vi "GOOP_ClassTool.vi"(0 "ClassRef":refnum<vi>, 5 "Error In":errorcluster) -> (19 "Error Out":errorcluster)   [LabVIEW 2014]
uses:
  <resource>/Framework/Providers/Open_GDS/ClassProviders/Common/ScriptingFunctions/Scripting_ConnectorPanePatternType.ctl
  <vilib>/regexp/Match Regular Expression.xnode
panel:
  out "ReasonWhyParentClassCan'tBeCreated 2":string
  in  "SelectAll":bool
  in  "ClassesCancel":bool
  in  "ClassesOK":bool
  in  "Classes":i32[](listbox)
  in  "MoreClasses":bool
  in  "Class(es)":u16(ring) items=["Oven", "-", "Equipment", "EquipmentVisitor", "GetCostVisitor", "Laser", "Oven", "PrintVisitor", "Rig"]
  in  "Tab":enum32{"CP", "ClassControlName", "Interface"}(tab)
  in  "ApplyCP":bool
  in  "CP2":u16(ring) caption="To" items=["4x4x4", "5x6x5", "6x8x6"]
  out "CP1":T1 caption="From" items=["4x4x4", "5x6x5", "6x8x6"]
  out "ClassNameOut":string
  out "ClassNameIn":string
  in  "ClassControlName":string(combo) caption="New names of class controls and indicators"
  in  "UpdateClassControlNames":bool
  in  "InterfaceToCreate":u16(ring) items=["Create a parent class based on some of my methods of my class: Oven", "Create an Interface(By VI Server) based on some of my methods of my class: Oven", "Create an Interface and Adaptor class based on some of my methods of my class: Oven"]
  out "InterfaceOptionTab":enum32{"Parent", "Adapter"}(tab)
  out "ReasonWhyParentClassCan'tBeCreated":string
  in  "CreateClassAndMethods":bool
  in  "ParentFolder":path
  in  "ParentClassName":string
  in  "ParentClass":u16(ring) items=["", "Equipment", "EquipmentVisitor", "GetCostVisitor", "Laser", "PrintVisitor", "Rig"]
  out "MyClassName(ParentClass)":string
  in  "MyClassMethods":i32[](listbox) caption="Class methods to add in the Interface class"
  out "Parent/InterafaceImage":u16(ring)
  out "MyClassName(InteraceClass)":string
  in  "InterfaceClassName 2":string
  in  "InterfaceFolder 2":path
  in  "Parent Methods":i32(listbox)
  in  "MyClassMethods(Interface)":i32[](listbox) caption="Class methods"
  in  "InterfaceClassName":string
  in  "InterfaceClass":u16(ring) items=["", "AbstractEdge", "Actor", "Last Ack", "Launch Nested Actor Msg", "Message", "Message Dequeuer", "Message Enqueuer", "Message Priority Queue", "Message Queue", "Stop Msg", "Actor1_BasicNoLib_G4_4.0.0", "Actor1_BasicNoLib_N_4.0.0", "Actor1_Basic_G4_4.0.0", "Actor1_Basic_N_4.0.0", "Actor1_GUI_G4_4.0.0", "StartMeasurement_Msg", "Actor1_GUI_N_4.0.0", "StartMeasurement_Msg", "AnotherClass", "ArrowHead", "Base", "BaseTemplate", "BaseTemplate_4x4x4", "BentStyle", "ByViServerInterfaceTemplate_4x4x4", "ByViServerInterfaceTemplate_6x8x6", "CallEdge", "ClassDiagramGraph", "ClassReader", "ClassReaderGOOP300", "ClassReaderGOOP400", "ClassReaderNative", "ClassRelationshipEdge", "ClassWriter", "ClassWriterGOOP300", "ClassWriterGOOP400", "ClassWriterNative", "DemoClass1", "DemoSubClass1", "DemoSubClass2", "DemoSubSubClass1", "Direction", "G4BaseTemplate_Simple_4x4x4", "G4BaseTemplate_Simple_6x8x6", "G4BaseTemplate_Singleton_4x4x4", "G4BaseTemplate_Singleton_6x8x6", "G4InterfaceTemplate_4x4x4", "G4InterfaceTemplate_6x8x6", "G4SubTemplate_Simple_4x4x4", "G4SubTemplate_Simple_6x8x6", "G4SubTemplate_Singleton_4x4x4", "G4SubTemplate_Singleton_6x8x6", "GOOP4_Base", "GOOP4_Sub", "GeneralPathEdge", "Graph", "Graphics", "Grid", "Interface1", "Leaf", "LineStyle", "Map", "Message_4.0.0", "MultiLineString", "NativeBaseTemplate", "NativeBaseTemplate_4x4x4", "NativeSubTemplate", "NativeSubTemplate_4x4x4", "NoteEdge", "Object", "Scripting", "SegmentedLineEdge", "SequenceDiagramGraph", "SingletonTemplate", "StateDiagramGraph", "StateReverse", "StateTransitionEdge", "Sub", "SubTemplate", "SubTemplate_4x4x4", "UmlEditor", "UseCaseDiagramGraph"]
  in  "InterfaceFolder":path
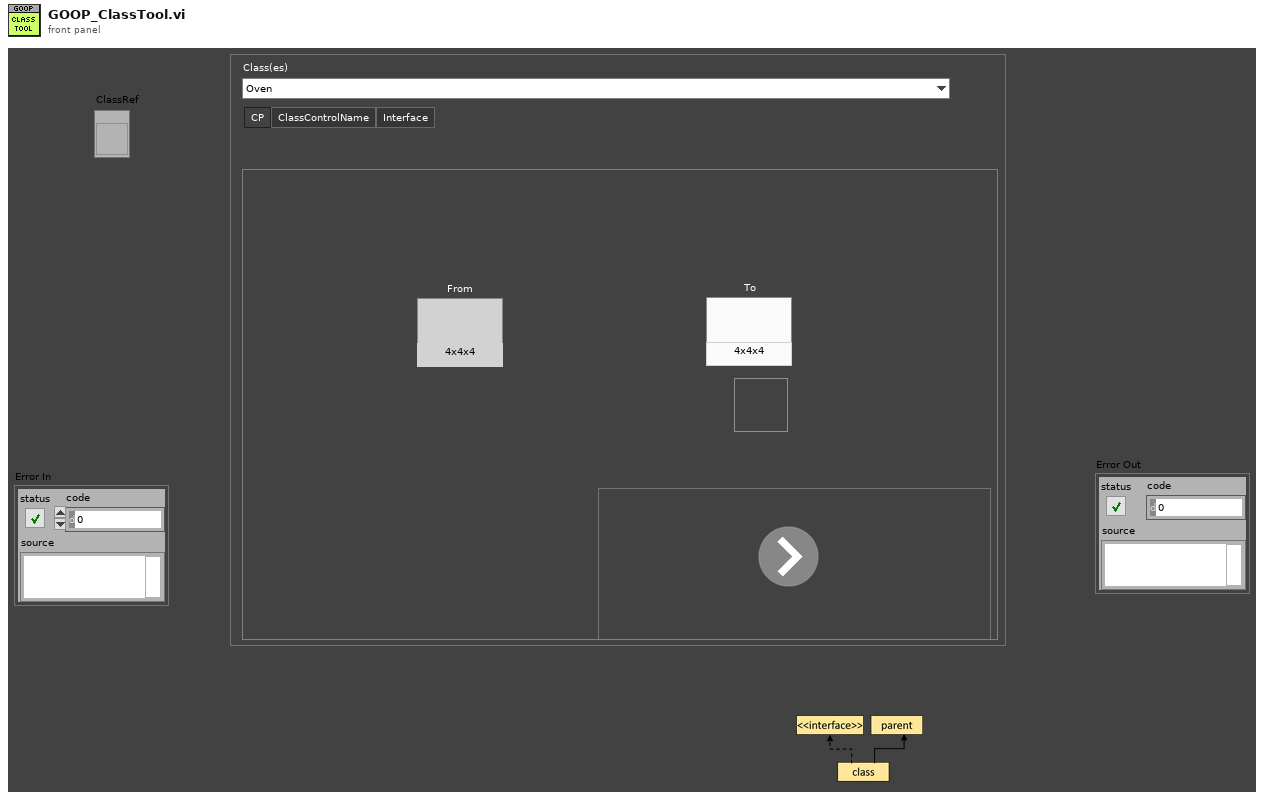
[diagram p1: front panel]
types:
  T1 = typedef "Scripting_ConnectorPanePatternType.ctl" = u16
  T2 = cluster{"Classes":refnum<vi>[], "Selected":i32[], "DropDownClasses":refnum<vi>[], "Interfaces":refnum<vi>[], "Methods":refnum<vi>[], "ParentClassIdx":i32}
  T3 = enum32{"Invalid", "Default", "Floating", "Floating/Auto-Hide", "Modal"}
  T4 = enum8{"Enabled", "Disabled", "Disabled and Grayed Out"}
  T5 = enum32{"invalid scope", "public", "private", "protected", "community"}
  T6 = typedef "GDSLvCLass_ClassSettingsType.ctl" = cluster{"ClassProviderName":string, "ClassTemplateUsed":string, "ClassTemplateVersion":string, "ClassDescription":string, "PlugIns":T7[], "ConnectorPanePattern":string}
  T7 = typedef "GDSLvClass_PlugIn.ctl" = cluster{"Type":T8, "ID":string, "Version":string, "Path":path, "Name":string, "Data":variant}
  T8 = typedef "GDSLvClass_PlugInTypes.ctl" = enum16{"DesignPattern", "MethodTypes"}
  T9 = cluster{"result string":string, "ClassRef":refnum<vi>}
  T10 = cluster{"result string":string, "ClassRef":refnum<vi>}[]
  T11 = typedef "lveventtype.ctl" = enum32{"Null", "Timeout", "Annotation Menu Selection", "Annotation Menu Selection?", "App Instance Close", "App Instance Close?", "Autoscale Range Change", "Bookmark Info Change", "Cell Edit", "Cell Edit?", "Cursor Grab", "Cursor Grab?", "Cursor Menu Selection", "Cursor Menu Selection?", "Cursor Move", "Cursor Release", "Data Change", "Direction Change", "Display State Change", "Drag Ended", "Drag Enter", "Drag Leave", "Drag Over", "Drag Source Update", "Drag Starting", "Drag Starting?", "Drop", "Exec State Change", "Key Down", "Key Down?", "Key Repeat", "Key Repeat?", "Key Up", "Listbox Double Click", "Menu Activation?", "Menu Selection (App)", "Menu Selection? (App)", "Menu Selection (User)", "Mouse Down", "Mouse Down?", "Mouse Enter", "Mouse Leave", "Mouse Move", "Mouse Up", "Mouse Wheel", "NI Security User Change (App)", "Pane Size", "Panel Close", "Panel Close?", "Panel Resize", "Plot Attribute Change", "Scale Range Change", "Shortcut Menu Activation?", "Shortcut Menu Selection (App)", "Shortcut Menu Selection? (App)", "Shortcut Menu Selection (User)", "Tree Double Click", "Tree Drag", "Tree Drag?", "Tree Drop", "Tree Drop?", "Tree Item Close", "Tree Item Close?", "Tree Item Open", "Tree Item Open?", "User Event", "Value Change"}
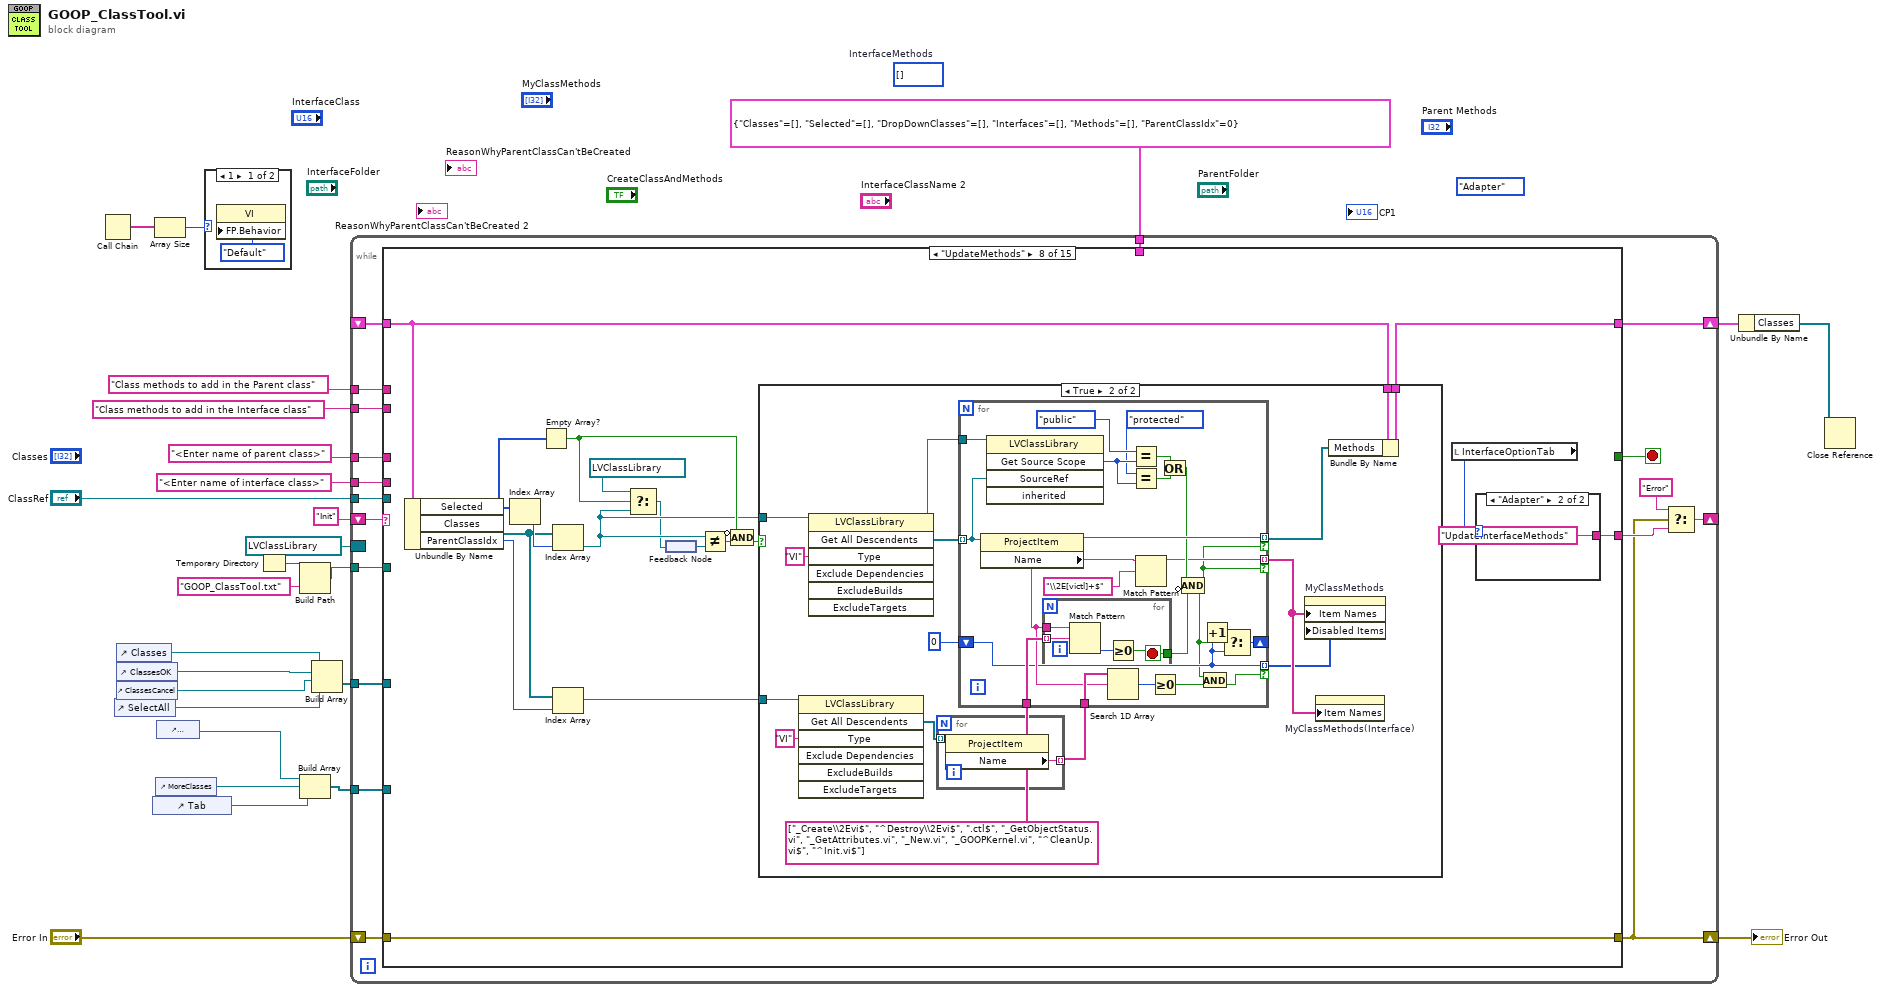
[diagram p0: block diagram]
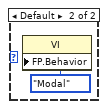
[diagram p2: hidden frame]
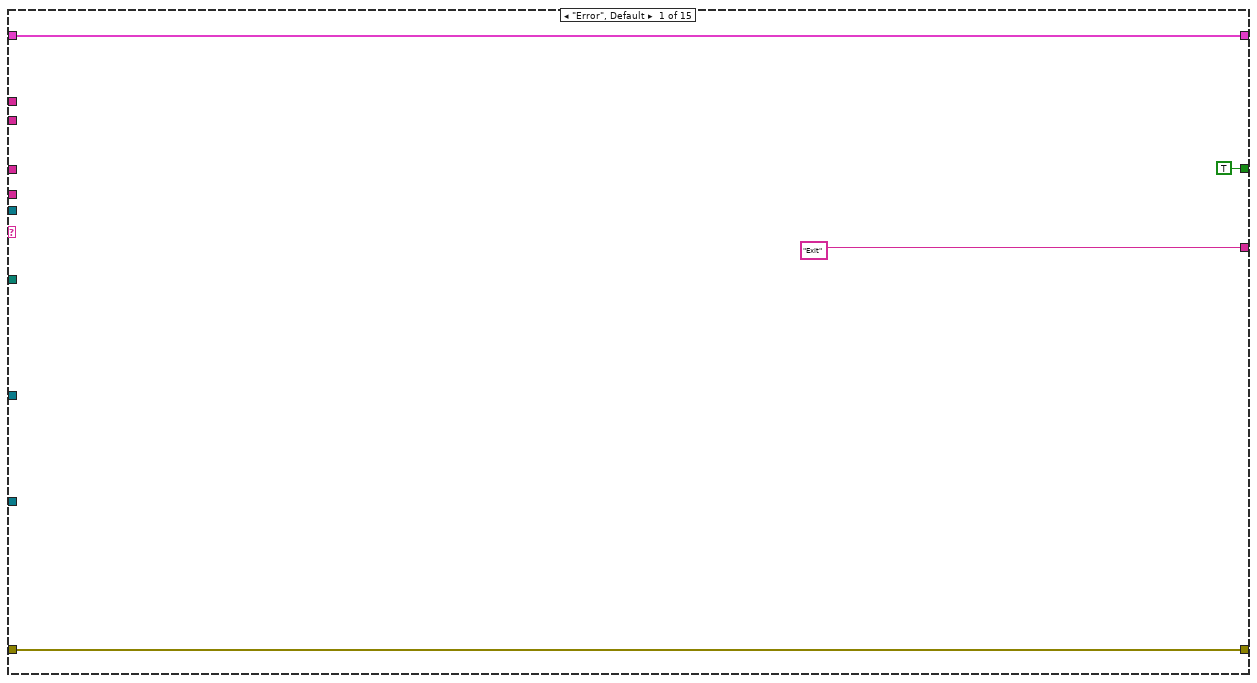
[diagram p3: hidden frame]
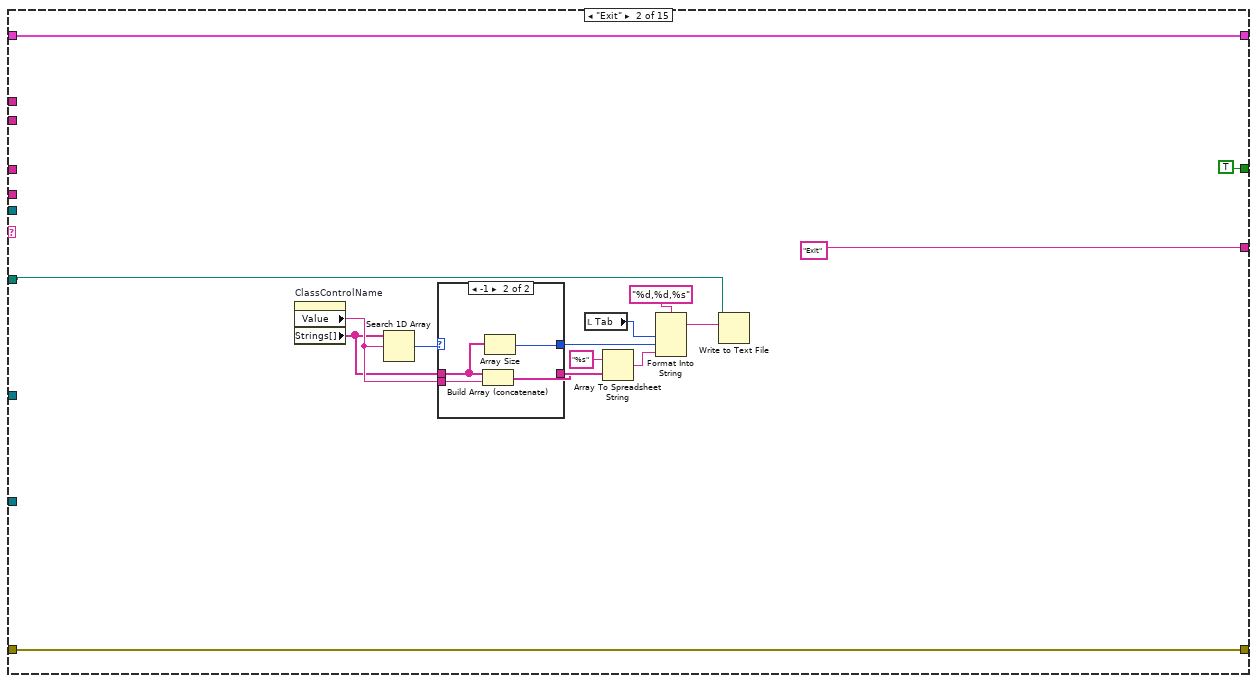
[diagram p4: hidden frame]
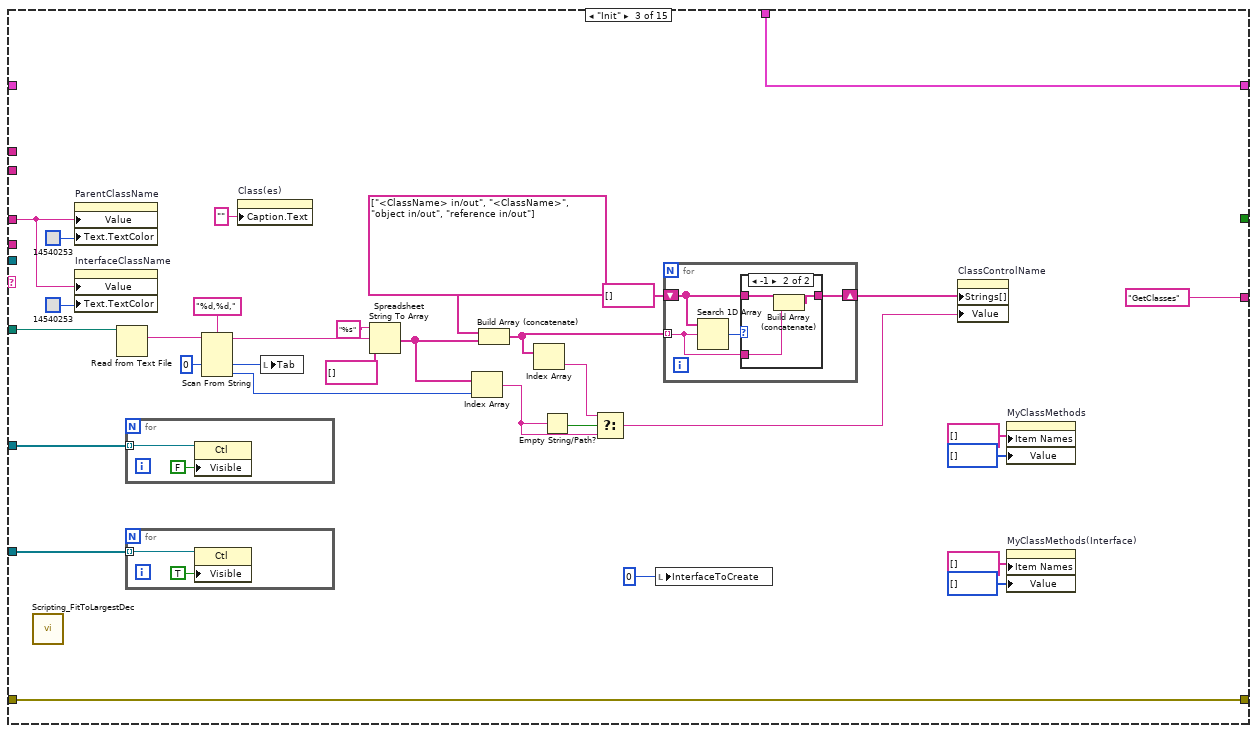
[diagram p6: hidden frame]
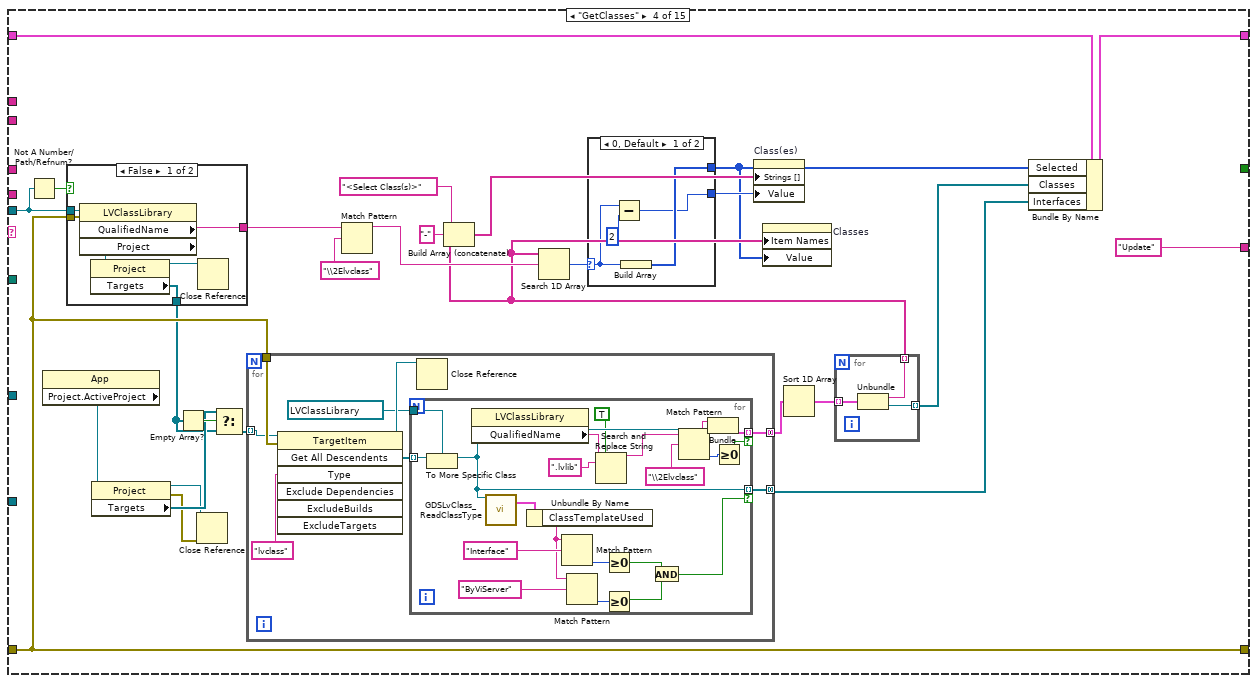
[diagram p8: hidden frame]
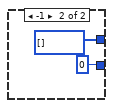
[diagram p9: hidden frame]
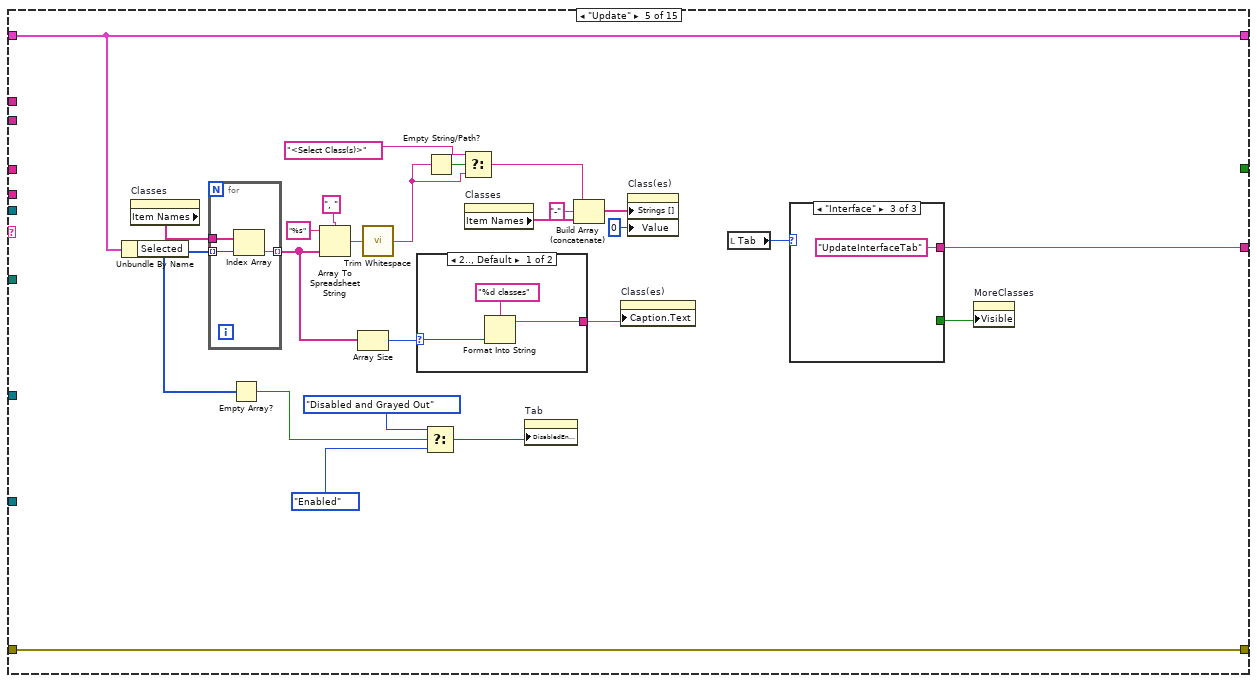
[diagram p11: hidden frame]
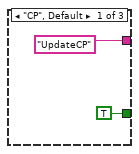
[diagram p12: hidden frame]
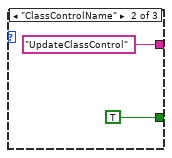
[diagram p13: hidden frame]
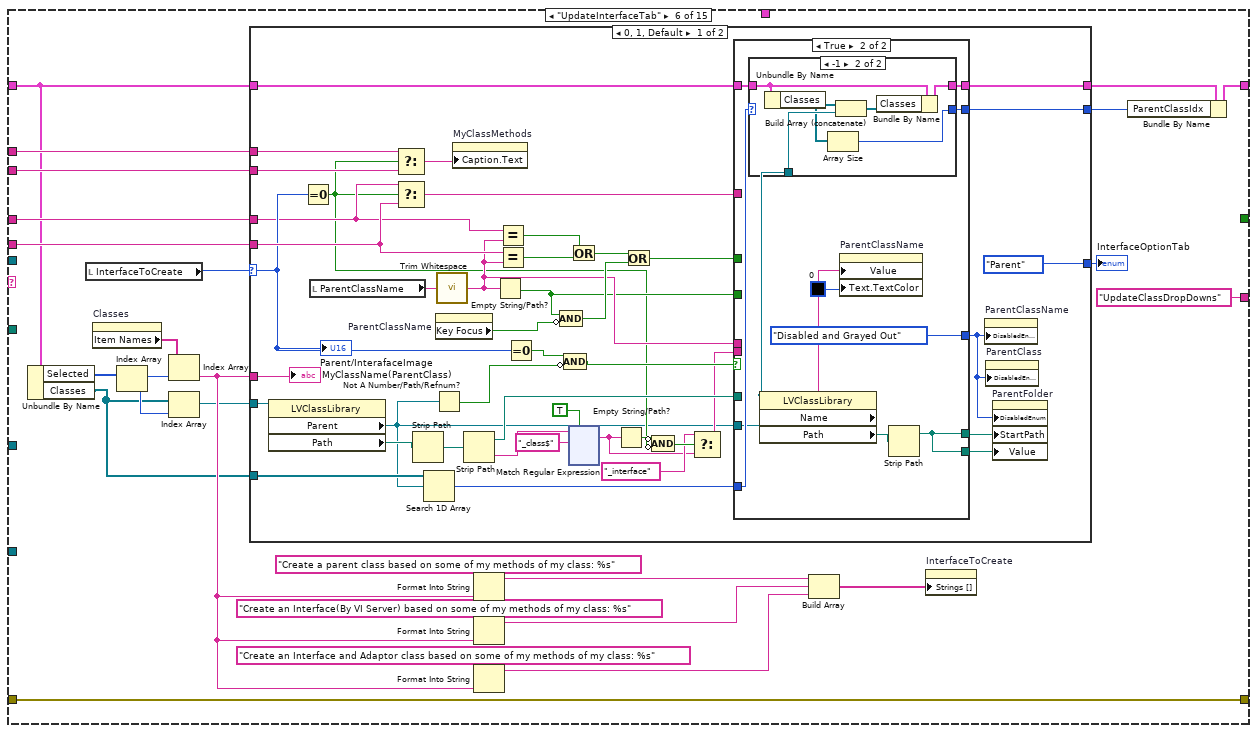
[diagram p15: hidden frame]
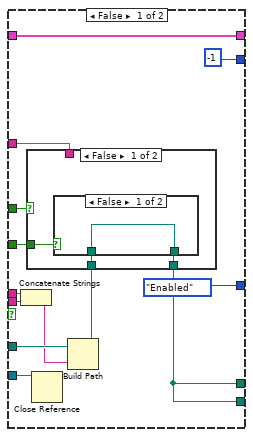
[diagram p16: hidden frame]
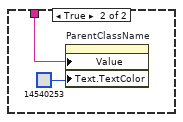
[diagram p18: hidden frame]
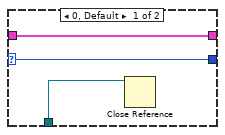
[diagram p19: hidden frame]
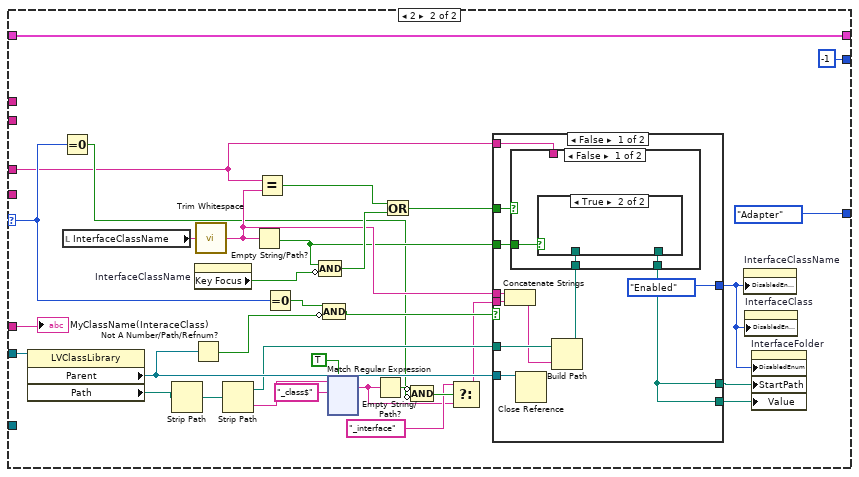
[diagram p20: hidden frame]
diagram:
  (unwired) enum32{"Parent", "Adapter"}."Adapter" ("InterfaceOptionTab")
  (unwired) i32[] []  # InterfaceMethods
  n1 = Call Chain() -> (call chain=w2:string[])
  n2 = control-ref of="SelectAll"() -> (w14:refnum<vi>)
  n3 = control-ref of="Classes"() -> (w23:refnum<vi>)
  n4 = control-ref of="ClassesOK"() -> (w22:refnum<vi>)
  n5 = control-ref of="ClassesCancel"() -> (w21:refnum<vi>)
  n6 = control-ref of="Tab"() -> (w18:refnum<vi>)
  n7 = Array Size(array=w2) -> (size(s)=w1:i32)
  n8 = control-ref of="MoreClasses"() -> (w19:refnum<vi>)
  n9 = control-ref of="Class(es)"() -> (w13:refnum<vi>)
  n10 = case shown="1" w1 {
    frame 1 {
      n11 = property class="VI"("FP.Behavior"=T3."Default" ("Front Panel Window:Behavior")) -> ()  [unwired: 2 in, 2 out]
    }
    frame Default {
      n12 = property class="VI"("FP.Behavior"=T3."Modal" ("Front Panel Window:Behavior")) -> ()  [unwired: 2 in, 2 out]
    }
  }
  n13 = Temporary Directory() -> (w9:path)
  n14 = Build Path(base path=w9, name or relative path="GOOP_ClassTool.txt") -> (appended path=w8:path)
  n15 = Build Array(w13, w19, w18) -> (w17:refnum<vi>[])
  n16 = Build Array(w23, w22, w21, w14) -> (w20:refnum<vi>[])
  n17 = while {
    shift-right: [w41] -> w24
    shift-left: "Error In" -> [w46]
    shift-right: [w44] -> _
    shift-left: "Init" -> [w45]
    shift-right: [w40] -> w12
    shift-left: _ -> [w39]
    tunnel: w20 -> [w38]
    tunnel: w17 -> [w37]
    tunnel: "ClassRef" -> [w36]
    tunnel: T2 {"Classes"=[], "Selected"=[], "DropDownClasses"=[], "Interfaces"=[], "Methods"=[], "ParentClassIdx"=0} -> [w35]
    tunnel: w8 -> [w34]
    tunnel: "<Enter name of parent class>" ("ParentClassName") -> [w32]
    tunnel: "<Enter name of interface class>" ("ParentClassName") -> [w31]
    tunnel: "Class methods to add in the Parent class" ("Caption.Text") -> [w30]
    tunnel: "Class methods to add in the Interface class" ("Caption.Text") -> [w29]
    border: refnum<vi> refnum ("ClassRef") -> [_]
    stop <- w33 stop-if-true
    n18 = case shown="\"UpdateMethods\"" w45 {
      tunnel: w46 -> [w50 w65 w102 w125 w212 w238 w619 w688 w736 w766 w814 w973 w982 w1000 w1042]
      tunnel: [w50 w65 w102 w125 w212 w238 w619 w688 w736 w766 w814 w973 w981 w997 w1042] -> w41
      tunnel: ["Exit" "Exit" "GetClasses" "Update" w200 "UpdateClassDropDowns" "UpdateMethods" w676 _ _ w815 "Update" "Exit" "Exit" _] -> w42
      tunnel: [w48 w63 w98 w128 w201 w227 w618 w684 w737 w765 w816 w974 w983 w1003 w1041] -> w40
      tunnel: w39 -> [w48 w63 _ w141 w201 w226 w616 w685 w737 w765 w811 w976 w983 w1003 w1041]
      tunnel: w38 -> [_ _ w101 _ _ _ _ _ _ _ w813 _ _ _ _]
      tunnel: w37 -> [_ _ w100 _ _ _ _ _ _ _ w812 _ _ _ _]
      tunnel: w36 -> [_ _ _ w124 _ _ _ _ _ _ _ _ _ _ _]
      tunnel: w35 -> [_ _ w98 _ _ _ _ _ _ _ _ _ _ _ _]
      tunnel: w34 -> [_ w52 w90 _ _ _ _ _ _ _ _ _ _ _ _]
      tunnel: [TRUE TRUE _ _ _ _ _ _ _ _ _ _ _ _ _] -> w33
      tunnel: w32 -> [_ _ w72 _ _ w237 _ _ _ _ w810 _ _ _ _]
      tunnel: w31 -> [_ _ _ _ _ w234 _ _ _ _ w808 _ _ _ _]
      tunnel: w30 -> [_ _ _ _ _ w230 _ _ _ _ _ _ _ _ _]
      tunnel: w29 -> [_ _ _ _ _ w229 _ _ _ _ _ _ _ _ _]
      frame "Error", Default {
      }
      frame "Exit" {
        n19 = property on="ClassControlName" class="CmbBox"() -> ("Value"=w57:string, "Strings[]"=w56:string[])  [unwired: 2 in, 2 out]
        n20 = Search 1D Array(1D array=w56, element=w57) -> (index of element=w53:i32)  [unwired: 1 in]
        n21 = case shown="-1" w53 {
          selector: w53 -> [w67 _]
          tunnel: [w67 w69] -> w54
          tunnel: w56 -> [w66 w70]
          tunnel: w57 -> [_ w71]
          tunnel: [w66 w68] -> w60
          frame 0, Default {
          }
          frame -1 {
            n22 = Build Array (concatenate)(w70, w71) -> (w68:string[])
            n23 = Array Size(array=w70) -> (size(s)=w69:i32)
          }
        }
        n24 = local read "Tab"() -> (w62:enum32{"CP", "ClassControlName", "Interface"})
        n25 = Array To Spreadsheet String(array=w60, 3:"%s" ("format string")) -> (spreadsheet string=w59:string)  [unwired: 1 in]
        n26 = Format Into String(format string="%d,%d,%s", w62, w54, w59) -> (resulting string=w61:string)  [unwired: 2 in, 1 out]
        n27 = Write to Text File(file (use dialog)=w52, text=w61) -> ()  [unwired: 2 in, 3 out]
      }
      frame "Init" {
        n28 = call <resource>:"Scripting_FitToLargestDec.vi"() -> ()  [unwired: 6 in, 2 out]
        n29 = property on="ParentClassName" class="Str"("Value"=w72, "Text.TextColor"=u32 14540253) -> ()  [unwired: 2 in, 2 out]
        n30 = property on="InterfaceClassName" class="Str"("Value"=w72, "Text.TextColor"=u32 14540253) -> ()  [unwired: 2 in, 2 out]
        n31 = Read from Text File(file (use dialog)=w90) -> (text=w97:string)  [unwired: 3 in, 3 out]
        n32 = for {
          tunnel: w101 -> [w115] mode=indexing
          n33 = property on="Property Node" class="Ctl"(reference=w115, "Visible"=FALSE) -> ()  [unwired: 1 in, 2 out]
        }
        n34 = for {
          tunnel: w100 -> [w113] mode=indexing
          n35 = property on="Property Node" class="Ctl"(reference=w113, "Visible"=TRUE) -> ()  [unwired: 1 in, 2 out]
        }
        n36 = Scan From String(format string="%d,%d,", input string=w97, default 1=0 ("default value 1")) -> (remaining string=w95:string, output 1=w88:i32, output 2=w86:i32)  [unwired: 3 in, 2 out]
        n37 = property on="Class(es)" class="Ring (strict)"("Caption.Text"="") -> ()  [unwired: 2 in, 2 out]
        n38 = local write "Tab"(w88) -> ()
        n39 = Spreadsheet String To Array(format string="%s", spreadsheet string=w95, array type (2D Dbl)=string[] []) -> (array=w87:string[])  [unwired: 1 in]
        n40 = Index Array(array=w87, index=w86) -> (element=w81:string)
        n41 = Build Array (concatenate)(string[] ["<ClassName> in/out", "<ClassName>", "object in/out", "reference in/out"] ("Strings []"), w87) -> (w84:string[])
        n42 = Index Array(array=w84) -> (element=w82:string)  [unwired: 1 in]
        n43 = Empty String/Path?(string/path=w81) -> (empty?=w83:bool)
        n44 = Select(t=w82, s=w83, f=w81) -> (s? t:f=w80:string)
        n45 = local write "InterfaceToCreate"(0) -> ()
        n46 = for {
          tunnel: w84 -> [w105] mode=indexing
          shift-right: [w104] -> w85
          shift-left: string[] [] -> [w106]
          n47 = Search 1D Array(1D array=w106, element=w105) -> (index of element=w107:i32)  [unwired: 1 in]
          n48 = case shown="-1" w107 {
            tunnel: w106 -> [w108 w111]
            tunnel: w105 -> [_ w110]
            tunnel: [w108 w109] -> w104
            frame 0, Default {
            }
            frame -1 {
              n49 = Build Array (concatenate)(w111, w110) -> (w109:string[])
            }
          }
        }
        n50 = property on="ClassControlName" class="CmbBox"("Strings[]"=w85, "Value"=w80) -> ()  [unwired: 2 in, 2 out]
        n51 = property on="MyClassMethods" class="LstBox (strict)"("Item Names"=string[] [], "Value"=i32[] [] ("MyClassMethods")) -> ()  [unwired: 2 in, 2 out]
        n52 = property on="MyClassMethods(Interface)" class="LstBox (strict)"("Item Names"=string[] [], "Value"=i32[] [] ("MyClassMethods")) -> ()  [unwired: 2 in, 2 out]
      }
      frame "GetClasses" {
        n53 = Not A Number/Path/Refnum?(number/path/refnum=w124) -> (NaN/Path/Refnum?=w123:bool)
        n54 = property class="App"() -> ("Project.ActiveProject"=w122:refnum<vi>)  [unwired: 2 in, 2 out]
        n55 = case shown="False" w123 {
          tunnel: [w154 _] -> w140
          tunnel: [w152 _] -> w121
          tunnel: w125 -> [w151 _]
          tunnel: w124 -> [w150 _]
          frame False {
            n56 = property class="LVClassLibrary"(reference=w150, error in=w151) -> ("QualifiedName"=w154:string, "Project"=w153:refnum<vi>)  [unwired: 2 out]
            n57 = property class="Project"(reference=w153) -> (reference out=w149:refnum<vi>, "Targets"=w152:refnum<vi>[])  [unwired: 1 in, 1 out]
            n58 = Close Reference(reference=w149) -> ()  [unwired: 1 in, 1 out]
          }
          frame True {
          }
        }
        n59 = property class="Project"(reference=w122) -> (reference out=w117:refnum<vi>, error out=w118:errorcluster, "Targets"=w133:refnum<vi>[])  [unwired: 1 in]
        n60 = Empty Array?(array=w121) -> (empty?=w134:bool)
        n61 = Close Reference(reference=w117, error in (no error)=w118) -> ()  [unwired: 1 out]
        n62 = Select(t=w133, s=w134, f=w121) -> (s? t:f=w132:refnum<vi>[])
        n63 = for {
          tunnel: [w163] -> w136 mode=concatenating
          tunnel: w125 -> [w162]
          tunnel: w132 -> [w161] mode=indexing
          tunnel: [w158] -> w116 mode=concatenating
          n64 = invoke class="TargetItem" method="Get All Descendents"(reference=w161, error in=w162, "Type"="lvclass") -> (reference out=w160:refnum<vi>, "All Descendents"=w164:refnum<vi>[])  [unwired: 4 in, 5 out]
          n65 = for {
            tunnel: w164 -> [w187] mode=indexing
            tunnel: [w181] -> w163 mode=indexing if=w184
            tunnel: refnum<vi> refnum ("ClassRef") -> [w176]
            tunnel: [w167] -> w158 mode=indexing if=w166
            n66 = To More Specific Class(target class=w176, reference=w187) -> (specific class reference=w167:refnum<vi>)  [unwired: 1 in, 1 out]
            n67 = property class="LVClassLibrary"(reference=w167) -> (reference out=w182:refnum<vi>, "QualifiedName"=w180:string)  [unwired: 1 in, 1 out]
            n68 = call <resource>:"GDSLvClass_ReadClassType.vi"("Class Refnum In"=w167) -> ("ClassSettings"=w173:T6)  [unwired: 16 in, 2 out]
            n69 = Unbundle By Name(w173) -> ("ClassTemplateUsed"=w170:string)
            n70 = Match Pattern(string=w170, regular expression="Interface") -> (offset past match=w171:i32)  [unwired: 1 in, 3 out]
            n71 = Match Pattern(string=w170, regular expression="ByViServer") -> (offset past match=w168:i32)  [unwired: 1 in, 3 out]
            n72 = Search and Replace String(replace all?=TRUE ("replace all? (F)"), input string=w180, search string=".lvlib" ("regular expression")) -> (result string=w179:string)  [unwired: 5 in, 3 out]
            n73 = Greater Or Equal To 0?(x=w171) -> (x >= 0?=w174:bool)
            n74 = Greater Or Equal To 0?(x=w168) -> (x >= 0?=w175:bool)
            n75 = And(x=w174, y=w175) -> (x .and. y?=w166:bool)
            n76 = Match Pattern(string=w179, regular expression="\\2Elvclass") -> (before substring=w183:string, offset past match=w185:i32)  [unwired: 1 in, 2 out]
            n77 = Bundle("result string"=w183, "ClassRef"=w182) -> (w181:T9)  [unwired: 1 in]
            n78 = Greater Or Equal To 0?(x=w185) -> (x >= 0?=w184:bool)
          }
          n79 = Close Reference(reference=w160) -> ()  [unwired: 1 in, 1 out]
        }
        n80 = Match Pattern(string=w140, regular expression="\\2Elvclass") -> (before substring=w131:string)  [unwired: 1 in, 3 out]
        n81 = Sort 1D Array(array=w136) -> (sorted array=w130:T10)
        n82 = for {
          tunnel: w130 -> [w157] mode=indexing
          tunnel: [w156] -> w127 mode=indexing
          tunnel: [w155] -> w129 mode=indexing
          n83 = Unbundle(w157) -> ("result string"=w155:string, "ClassRef"=w156:refnum<vi>)
        }
        n84 = Build Array (concatenate)("<Select Class(s)>" ("element"), "-" ("element"), w129) -> (w137:string[])
        n85 = Search 1D Array(1D array=w129, element=w131) -> (index of element=w120:i32)  [unwired: 1 in]
        n86 = case shown="0, Default" w120 {
          selector: w120 -> [w146 _]
          tunnel: [w143 0 ("Classes")] -> w135
          tunnel: [w145 i32[] [] ("Classes")] -> w119
          frame 0, Default {
            n87 = Subtract(x=w146, y=2) -> (x-y=w143:i32)
            n88 = Build Array(w146) -> (w145:i32[])
          }
          frame -1 {
          }
        }
        n89 = property on="Class(es)" class="Ring (strict)"("Strings []"=w137, "Value"=w135) -> ()  [unwired: 2 in, 2 out]
        n90 = property on="Classes" class="LstBox (strict)"("Item Names"=w129, "Value"=w119) -> ()  [unwired: 2 in, 2 out]
        n91 = Bundle By Name(cluster=w141, "Selected"=w119, "Classes"=w127, "Interfaces"=w116) -> (w128:T2)
      }
      frame "Update" {
        n92 = Unbundle By Name(w201) -> ("Selected"=w199:i32[])
        n93 = property on="Classes" class="LstBox (strict)"() -> ("Item Names"=w211:string[])  [unwired: 2 in, 2 out]
        n94 = for {
          tunnel: w199 -> [w223] mode=indexing
          tunnel: w211 -> [w222]
          tunnel: [w221] -> w188 mode=indexing
          n95 = Index Array(array=w222, index=w223) -> (element=w221:string)
        }
        n96 = Empty Array?(array=w199) -> (empty?=w198:bool)
        n97 = Array To Spreadsheet String(delimiter (Tab)=", ", array=w188, 3:"%s" ("format string")) -> (spreadsheet string=w208:string)
        n98 = Array Size(array=w188) -> (size(s)=w207:i32)
        n99 = call <vilib>:"Trim Whitespace.vi"("string"=w208) -> ("trimmed string"=w192:string)  [unwired: 1 in]
        n100 = case shown="2.., Default" w207 {
          selector: w207 -> [w220 _]
          tunnel: [w218 _] -> w206
          frame 2.., Default {
            n101 = Format Into String(format string="%d classes", w220) -> (resulting string=w218:string)  [unwired: 2 in, 1 out]
          }
          frame ..1 {
          }
        }
        n102 = Select(t=T4."Disabled and Grayed Out", s=w198, f=T4."Enabled" ("Disabled")) -> (s? t:f=w195:T4)
        n103 = Empty String/Path?(string/path=w192) -> (empty?=w194:bool)
        n104 = Select(t="<Select Class(s)>" ("element"), s=w194, f=w192) -> (s? t:f=w191:string)
        n105 = property on="Classes" class="LstBox (strict)"() -> ("Item Names"=w205:string[])  [unwired: 2 in, 2 out]
        n106 = property on="Tab" class="TabCtl (strict)"("DisabledEnum"=w195) -> ()  [unwired: 2 in, 2 out]
        n107 = Build Array (concatenate)(w191, "-" ("element"), w205) -> (w204:string[])
        n108 = property on="Class(es)" class="Ring (strict)"("Caption.Text"=w206) -> ()  [unwired: 2 in, 2 out]
        n109 = property on="Class(es)" class="Ring (strict)"("Strings []"=w204, "Value"=0 ("Classes")) -> ()  [unwired: 2 in, 2 out]
        n110 = local read "Tab"() -> (w190:enum32{"CP", "ClassControlName", "Interface"})
        n111 = case shown="\"Interface\"" w190 {
          tunnel: ["UpdateCP" "UpdateClassControl" "UpdateInterfaceTab"] -> w200
          tunnel: [TRUE TRUE _] -> w189
          frame "CP", Default {
          }
          frame "ClassControlName" {
          }
          frame "Interface" {
          }
        }
        n112 = property on="MoreClasses" class="Bool"("Visible"=w189) -> ()  [unwired: 2 in, 2 out]
      }
      frame "UpdateInterfaceTab" {
        n113 = Unbundle By Name(w226) -> ("Selected"=w248:i32[], "Classes"=w228:refnum<vi>[])
        n114 = local read "InterfaceToCreate"() -> (w235:u16)
        n115 = property on="Classes" class="LstBox (strict)"() -> ("Item Names"=w247:string[])  [unwired: 2 in, 2 out]
        n116 = Index Array(array=w248) -> (element=w232:i32)  [unwired: 1 in]
        n117 = Index Array(array=w247, index=w232) -> (element=w239:string)
        n118 = Index Array(array=w228, index=w232) -> (element=w231:refnum<vi>)
        n119 = case shown="0, 1, Default" w235 {
          selector: w235 -> [w278 w468]
          tunnel: w239 -> [w291 w448]
          tunnel: w237 -> [w266 w447]
          tunnel: [enum32{"Parent", "Adapter"}."Parent" ("InterfaceOptionTab") enum32{"Parent", "Adapter"}."Adapter" ("InterfaceOptionTab")] -> w236
          tunnel: w234 -> [w283 _]
          tunnel: w231 -> [w281 w472]
          tunnel: w230 -> [w265 _]
          tunnel: w229 -> [w264 _]
          tunnel: w228 -> [w254 _]
          tunnel: w226 -> [w251 w445]
          tunnel: [w250 w445] -> w225
          tunnel: [w249 -1 ("index of element")] -> w224
          frame 0, 1, Default {
            n120 = property class="LVClassLibrary"(reference=w281) -> ("Parent"=w253:refnum<vi>, "Path"=w275:path)  [unwired: 1 in, 2 out]
            n121 = Equal To 0?(x=w278) -> (x = 0?=w260:bool)
            n122 = local read "ParentClassName"() -> (w290:string)
            n123 = Select(t=w265, s=w260, f=w264) -> (s? t:f=w263:string)
            n124 = Select(t=w266, s=w260, f=w283) -> (s? t:f=w282:string)
            n125 = Strip Path(path=w275) -> (stripped path=w274:path)  [unwired: 1 out]
            n126 = Search 1D Array(1D array=w254, element=w253) -> (index of element=w252:i32)  [unwired: 1 in]
            n127 = Not A Number/Path/Refnum?(number/path/refnum=w253) -> (NaN/Path/Refnum?=w279:bool)
            n128 = property on="ParentClassName" class="Str"() -> ("Key Focus"=w289:bool)  [unwired: 2 in, 2 out]
            n129 = call <vilib>:"Trim Whitespace.vi"("string"=w290) -> ("trimmed string"=w268:string)  [unwired: 1 in]
            n130 = property on="MyClassMethods" class="LstBox (strict)"("Caption.Text"=w263) -> ()  [unwired: 2 in, 2 out]
            n131 = Strip Path(path=w274) -> (stripped path=w267:path, name=w271:string)
            n132 = Empty String/Path?(string/path=w268) -> (empty?=w262:bool)
            n133 = Equal?(x=w266, y=w268) -> (x = y?=w285:bool)
            n134 = Equal?(x=w283, y=w268) -> (x = y?=w286:bool)
            n135 = Equal To 0?(x=w278) -> (x = 0?=w277:bool)
            n136 = Compound Arithmetic op=AND(w262, invert w289) -> (w288:bool)
            n137 = Compound Arithmetic op=AND(w277, invert w279) -> (w276:bool)
            n138 = Or(x=w285, y=w286) -> (x .or. y?=w284:bool)
            n139 = xnode "Match Regular Expression"("input string"=w271, "regular expression"="_class$", "ignore case? (F)"=TRUE) -> ("whole match"=w257:string)  [unwired: 3 in, 4 out]
            n140 = Empty String/Path?(string/path=w257) -> (empty?=w261:bool)
            n141 = Or(x=w284, y=w288) -> (x .or. y?=w280:bool)
            n142 = Compound Arithmetic op=AND(invert w261, invert w260) -> (w259:bool)
            n143 = Select(t="_interface" ("regular expression"), s=w259, f=w257) -> (s? t:f=w256:string)
            n144 = case shown="True" w276 {
              tunnel: w282 -> [w418 _]
              tunnel: w253 -> [w416 w426]
              tunnel: w280 -> [w417 _]
              tunnel: [T4."Enabled" ("Disabled") T4."Disabled and Grayed Out" ("Disabled")] -> w255
              tunnel: [w410 w430] -> w273
              tunnel: [w410 w430] -> w272
              tunnel: w268 -> [w415 _]
              tunnel: w256 -> [w414 _]
              tunnel: w267 -> [w413 _]
              tunnel: w262 -> [w408 _]
              tunnel: w252 -> [_ w429]
              tunnel: w251 -> [w407 w428]
              tunnel: [w407 w427] -> w250
              tunnel: [-1 ("index of element") w425] -> w249
              frame False {
                n145 = Concatenate Strings(w415, w414) -> (w412:string)
                n146 = Close Reference(reference=w416) -> ()  [unwired: 1 in, 1 out]
                n147 = Build Path(base path=w413, name or relative path=w412) -> (appended path=w411:path)
                n148 = case shown="False" w417 {
                  tunnel: w418 -> [_ w423]
                  tunnel: w411 -> [w420 _]
                  tunnel: [w419 _] -> w410
                  tunnel: w408 -> [w421 _]
                  frame False {
                    n149 = case shown="False" w421 {
                      tunnel: w420 -> [w422 _]
                      tunnel: [w422 _] -> w419
                      frame False {
                      }
                      frame True {
                      }
                    }
                  }
                  frame True {
                    n150 = property on="ParentClassName" class="Str"("Value"=w423, "Text.TextColor"=u32 14540253) -> ()  [unwired: 2 in, 2 out]
                  }
                }
              }
              frame True {
                n151 = case shown="-1" w429 {
                  selector: w429 -> [w435 _]
                  tunnel: w428 -> [w437 w442]
                  tunnel: [w437 w443] -> w427
                  tunnel: w426 -> [w436 w440]
                  tunnel: [w435 w438] -> w425
                  frame 0, Default {
                    n152 = Close Reference(reference=w436) -> ()  [unwired: 1 in, 1 out]
                  }
                  frame -1 {
                    n153 = Unbundle By Name(w442) -> ("Classes"=w439:refnum<vi>[])
                    n154 = Array Size(array=w439) -> (size(s)=w438:i32)
                    n155 = Build Array (concatenate)(w439, w440) -> (w441:refnum<vi>[])
                    n156 = Bundle By Name(cluster=w442, "Classes"=w441) -> (w443:T2)
                  }
                }
                n157 = property class="LVClassLibrary"(reference=w426) -> ("Name"=w432:string, "Path"=w431:path)  [unwired: 1 in, 2 out]
                n158 = property on="ParentClassName" class="Str"("Value"=w432, "Text.TextColor"=u32 0) -> ()  [unwired: 2 in, 2 out]
                n159 = Strip Path(path=w431) -> (stripped path=w430:path)  [unwired: 1 out]
              }
            }
            n160 = property on="ParentClassName" class="Str"("DisabledEnum"=w255) -> ()  [unwired: 2 in, 2 out]
            n161 = property on="ParentClass" class="Ring (strict)"("DisabledEnum"=w255) -> ()  [unwired: 2 in, 2 out]
            n162 = property on="ParentFolder" class="Path"("DisabledEnum"=w255, "StartPath"=w273, "Value"=w272) -> ()  [unwired: 2 in, 2 out]
            "MyClassName(ParentClass)" <- w291
            "Parent/InterafaceImage" <- w278
          }
          frame 2 {
            n163 = property class="LVClassLibrary"(reference=w472) -> ("Parent"=w471:refnum<vi>, "Path"=w465:path)  [unwired: 1 in, 2 out]
            n164 = Equal To 0?(x=w468) -> (x = 0?=w454:bool)
            n165 = local read "InterfaceClassName"() -> (w476:string)
            n166 = Strip Path(path=w465) -> (stripped path=w464:path)  [unwired: 1 out]
            n167 = Not A Number/Path/Refnum?(number/path/refnum=w471) -> (NaN/Path/Refnum?=w469:bool)
            n168 = property on="InterfaceClassName" class="Str"() -> ("Key Focus"=w475:bool)  [unwired: 2 in, 2 out]
            n169 = call <vilib>:"Trim Whitespace.vi"("string"=w476) -> ("trimmed string"=w458:string)  [unwired: 1 in]
            n170 = Strip Path(path=w464) -> (stripped path=w457:path, name=w461:string)
            n171 = Empty String/Path?(string/path=w458) -> (empty?=w456:bool)
            n172 = Equal?(x=w447, y=w458) -> (x = y?=w446:bool)
            n173 = Equal To 0?(x=w468) -> (x = 0?=w467:bool)
            n174 = Compound Arithmetic op=AND(w456, invert w475) -> (w474:bool)
            n175 = Compound Arithmetic op=AND(w467, invert w469) -> (w466:bool)
            n176 = xnode "Match Regular Expression"("input string"=w461, "regular expression"="_class$", "ignore case? (F)"=TRUE) -> ("whole match"=w451:string)  [unwired: 3 in, 4 out]
            n177 = Empty String/Path?(string/path=w451) -> (empty?=w455:bool)
            n178 = Or(x=w446, y=w474) -> (x .or. y?=w470:bool)
            n179 = Compound Arithmetic op=AND(invert w455, invert w454) -> (w453:bool)
            n180 = Select(t="_interface" ("regular expression"), s=w453, f=w451) -> (s? t:f=w450:string)
            n181 = case shown="False" w466 {
              tunnel: w447 -> [w601 _]
              tunnel: w471 -> [w599 w613]
              tunnel: w470 -> [w600 _]
              tunnel: [T4."Enabled" ("Disabled") T4."Disabled and Grayed Out" ("Disabled")] -> w449
              tunnel: [w593 w608] -> w463
              tunnel: [w593 w608] -> w462
              tunnel: w458 -> [w598 _]
              tunnel: w450 -> [w597 _]
              tunnel: w457 -> [w596 _]
              tunnel: w456 -> [w591 _]
              frame False {
                n182 = Concatenate Strings(w598, w597) -> (w595:string)
                n183 = Close Reference(reference=w599) -> ()  [unwired: 1 in, 1 out]
                n184 = Build Path(base path=w596, name or relative path=w595) -> (appended path=w594:path)
                n185 = case shown="False" w600 {
                  tunnel: w601 -> [_ w606]
                  tunnel: w594 -> [w603 _]
                  tunnel: [w602 _] -> w593
                  tunnel: w591 -> [w604 _]
                  frame False {
                    n186 = case shown="True" w604 {
                      tunnel: w603 -> [w605 _]
                      tunnel: [w605 _] -> w602
                      frame False {
                      }
                      frame True {
                      }
                    }
                  }
                  frame True {
                    n187 = property on="InterfaceClassName" class="Str"("Value"=w606, "Text.TextColor"=u32 14540253) -> ()  [unwired: 2 in, 2 out]
                  }
                }
              }
              frame True {
                n188 = property class="LVClassLibrary"(reference=w613) -> (reference out=w614:refnum<vi>, "Name"=w610:string, "Path"=w609:path)  [unwired: 1 in, 1 out]
                n189 = property on="InterfaceClassName" class="Str"("Value"=w610, "Text.TextColor"=u32 0) -> ()  [unwired: 2 in, 2 out]
                n190 = Strip Path(path=w609) -> (stripped path=w608:path)  [unwired: 1 out]
                n191 = Close Reference(reference=w614) -> ()  [unwired: 1 in, 1 out]
              }
            }
            n192 = property on="InterfaceClassName" class="Str"("DisabledEnum"=w449) -> ()  [unwired: 2 in, 2 out]
            n193 = property on="InterfaceClass" class="Ring (strict)"("DisabledEnum"=w449) -> ()  [unwired: 2 in, 2 out]
            n194 = property on="InterfaceFolder" class="Path"("DisabledEnum"=w449, "StartPath"=w463, "Value"=w462) -> ()  [unwired: 2 in, 2 out]
            "MyClassName(InteraceClass)" <- w448
          }
        }
        "InterfaceOptionTab" <- w236
        n195 = Format Into String(format string="Create a parent class based on some of my methods of my class: %s", w239) -> (resulting string=w245:string)  [unwired: 2 in, 1 out]
        n196 = Format Into String(format string="Create an Interface(By VI Server) based on some of my methods of my class: %s", w239) -> (resulting string=w242:string)  [unwired: 2 in, 1 out]
        n197 = Format Into String(format string="Create an Interface and Adaptor class based on some of my methods of my class: %s", w239) -> (resulting string=w240:string)  [unwired: 2 in, 1 out]
        n198 = Build Array(w245, w242, w240) -> (w244:string[])
        n199 = property on="InterfaceToCreate" class="Ring (strict)"("Strings []"=w244) -> ()  [unwired: 2 in, 2 out]
        n200 = Bundle By Name(cluster=w225, "ParentClassIdx"=w224) -> (w227:T2)
      }
      frame "UpdateClassDropDowns" {
        n201 = local read "InterfaceToCreate"() -> (w620:u16)
        n202 = case shown="0, Default" w620 {
          tunnel: [w627 w664] -> w617
          tunnel: w616 -> [w623 w665]
          frame 0, Default {
            n203 = Unbundle By Name(w623) -> ("Classes"=w622:refnum<vi>[], "Selected"=w621:i32[])
            n204 = Index Array(array=w621) -> (element=w624:i32)  [unwired: 1 in]
            n205 = Index Array(array=w622, index=w624) -> (element=w629:refnum<vi>)
            n206 = property class="LVClassLibrary"(reference=w629) -> ("Name"=w631:string)  [unwired: 1 in, 2 out]
            n207 = for {
              tunnel: w622 -> [w645] mode=indexing
              tunnel: w631 -> [w640]
              shift-right: [w636] -> w627
              shift-left: refnum<vi>[] [] -> [w638]
              n208 = property class="LVClassLibrary"(reference=w645) -> (reference out=w637:refnum<vi>, "Name"=w643:string)  [unwired: 1 in, 1 out]
              n209 = Build Array(w643) -> (w642:string[])
              n210 = while {
                shift-right: [w652] -> w644
                shift-left: w637 -> [w658]
                shift-right: [w653] -> w641
                shift-left: w642 -> [w655]
                i -> [w650]
                stop <- w656 stop-if-true
                n211 = property class="LVClassLibrary"(reference=w658) -> (reference out=w651:refnum<vi>, error out=w657:errorcluster, "Parent"=w652:refnum<vi>)  [unwired: 1 in]
                n212 = case shown="1.." w650 {
                  tunnel: w651 -> [_ w659]
                  frame Default {
                  }
                  frame 1.. {
                    n213 = Close Reference(reference=w659) -> ()  [unwired: 1 in, 1 out]
                  }
                }
                n214 = property class="LVClassLibrary"(reference=w652, error in=w657) -> (error out=w656:errorcluster, "Name"=w654:string)  [unwired: 1 out]
                n215 = case shown="No Error" w656 {
                  tunnel: w655 -> [w662 w663]
                  tunnel: w654 -> [w661 _]
                  tunnel: [w660 w663] -> w653
                  frame No Error {
                    n216 = Build Array (concatenate)(w662, w661) -> (w660:string[])
                  }
                  frame Error {
                  }
                }
              }
              n217 = Close Reference(reference=w644) -> ()  [unwired: 1 in, 1 out]
              n218 = Search 1D Array(1D array=w641, element=w640) -> (index of element=w639:i32)  [unwired: 1 in]
              n219 = case shown="0, Default" w639 {
                tunnel: w638 -> [w646 w649]
                tunnel: w637 -> [_ w648]
                tunnel: [w646 w647] -> w636
                frame 0, Default {
                }
                frame -1 {
                  n220 = Build Array (concatenate)(w649, w648) -> (w647:refnum<vi>[])
                }
              }
            }
            n221 = for {
              tunnel: w627 -> [w635] mode=indexing
              tunnel: [w632] -> w628 mode=indexing
              n222 = property class="LVClassLibrary"(reference=w635) -> ("Name"=w633:string)  [unwired: 1 in, 2 out]
              n223 = Match Pattern(string=w633, regular expression="\\2Elvclass") -> (before substring=w632:string)  [unwired: 1 in, 3 out]
            }
            n224 = Build Array (concatenate)("" ("regular expression"), w628) -> (w626:string[])
            n225 = property on="ParentClass" class="Ring (strict)"("Strings []"=w626) -> ()  [unwired: 2 in, 2 out]
          }
          frame 1 {
            n226 = Unbundle By Name(w665) -> ("Interfaces"=w664:refnum<vi>[])
            n227 = for {
              tunnel: w664 -> [w672] mode=indexing
              tunnel: [w669] -> w668 mode=indexing
              n228 = property class="LVClassLibrary"(reference=w672) -> ("Name"=w670:string)  [unwired: 1 in, 2 out]
              n229 = Match Pattern(string=w670, regular expression="\\2Elvclass") -> (before substring=w669:string)  [unwired: 1 in, 3 out]
            }
            n230 = Build Array (concatenate)("" ("regular expression"), w668) -> (w667:string[])
            n231 = property on="ParentClass" class="Ring (strict)"("Strings []"=w667) -> ()  [unwired: 2 in, 2 out]
          }
        }
        n232 = Bundle By Name(cluster=w616, "DropDownClasses"=w617) -> (w618:T2)
      }
      frame "UpdateMethods" {
        n233 = Unbundle By Name(w685) -> ("Selected"=w682:i32[], "Classes"=w675:refnum<vi>[], "ParentClassIdx"=w674:i32)
        n234 = Index Array(array=w682) -> (element=w689:i32)  [unwired: 1 in]
        n235 = Empty Array?(array=w682) -> (empty?=w681:bool)
        n236 = Index Array(array=w675, index=w689) -> (element=w680:refnum<vi>)
        n237 = Index Array(array=w675, index=w674) -> (element=w673:refnum<vi>)
        n238 = Select(t=refnum<vi> refnum, s=w681, f=w680) -> (s? t:f=w679:refnum<vi>)
        n239 = feedback-in #1(w679) -> ()
        n240 = feedback #1() -> (w687:refnum<vi>)
        n241 = Not Equal?(x=w680, y=w687) -> (x != y?=w686:bool)
        n242 = Compound Arithmetic op=AND(invert w681, w686) -> (w683:bool)
        n243 = case shown="True" w683 {
          tunnel: w680 -> [_ w700]
          tunnel: w685 -> [w691 w704]
          tunnel: [w691 w702] -> w684
          tunnel: w673 -> [_ w696]
          frame False {
          }
          frame True {
            n244 = invoke class="LVClassLibrary" method="Get All Descendents"(reference=w696, "Type"="VI") -> ("All Descendents"=w695:refnum<vi>[])  [unwired: 5 in, 6 out]
            n245 = invoke class="LVClassLibrary" method="Get All Descendents"(reference=w700, "Type"="VI") -> (reference out=w699:refnum<vi>, "All Descendents"=w705:refnum<vi>[])  [unwired: 5 in, 5 out]
            n246 = for {
              tunnel: w695 -> [w708] mode=indexing
              tunnel: [w707] -> w694 mode=indexing
              n247 = property class="ProjectItem"(reference=w708) -> ("Name"=w707:string)  [unwired: 1 in, 2 out]
            }
            n248 = for {
              tunnel: w705 -> [w727] mode=indexing
              tunnel: [w730] -> w703 mode=indexing if=w709
              tunnel: [w719] -> w698 mode=indexing if=w709
              tunnel: string[] ["_Create\\2Evi$", "^Destroy\\2Evi$", ".ctl$", "_GetObjectStatus.vi", "_GetAttributes.vi", "_New.vi", "_GOOPKernel.vi", "^CleanUp.vi$", "^Init.vi$"] -> [w729]
              tunnel: w699 -> [w728]
              tunnel: w694 -> [w717]
              shift-right: [w714] -> _
              shift-left: 0 -> [w712]
              tunnel: [w712] -> w692 mode=indexing if=w710
              n249 = property class="ProjectItem"(reference=w727) -> (reference out=w730:refnum<vi>, "Name"=w716:string)  [unwired: 1 in, 1 out]
              n250 = invoke class="LVClassLibrary" method="Get Source Scope"(reference=w728, "SourceRef"=w727) -> ("GetSourceScope"=w725:T5)  [unwired: 3 in, 4 out]
              n251 = for {
                tunnel: w716 -> [w734]
                tunnel: [w732] -> w721
                tunnel: w729 -> [w731] mode=indexing
                stop <- w732 stop-if-true
                n252 = Match Pattern(string=w734, regular expression=w731) -> (offset past match=w733:i32)  [unwired: 1 in, 3 out]
                n253 = Greater Or Equal To 0?(x=w733) -> (x >= 0?=w732:bool)
              }
              n254 = Search 1D Array(1D array=w717, element=w716) -> (index of element=w715:i32)  [unwired: 1 in]
              n255 = Equal?(x=T5."public" ("Source Scope:Get"), y=w725) -> (x = y?=w723:bool)
              n256 = Equal?(x=T5."protected" ("Source Scope:Get"), y=w725) -> (x = y?=w722:bool)
              n257 = Match Pattern(string=w716, regular expression="\\2E[victl]+$") -> (before substring=w719:string)  [unwired: 1 in, 3 out]
              n258 = Greater Or Equal To 0?(x=w715) -> (x >= 0?=w711:bool)
              n259 = Or(x=w723, y=w722) -> (x .or. y?=w720:bool)
              n260 = Compound Arithmetic op=AND(w720, invert w721) -> (w709:bool)
              n261 = And(x=w709, y=w711) -> (x .and. y?=w710:bool)
              n262 = Increment(x=w712) -> (x+1=w713:i32)
              n263 = Select(t=w713, s=w709, f=w712) -> (s? t:f=w714:i32)
            }
            n264 = property on="MyClassMethods" class="LstBox (strict)"("Item Names"=w698, "Disabled Items"=w692) -> ()  [unwired: 2 in, 2 out]
            n265 = property on="MyClassMethods(Interface)" class="LstBox (strict)"("Item Names"=w698) -> ()  [unwired: 2 in, 2 out]
            n266 = Bundle By Name(cluster=w704, "Methods"=w703) -> (w702:T2)
          }
        }
        n267 = local read "InterfaceOptionTab"() -> (w677:enum32{"Parent", "Adapter"})
        n268 = case shown="\"Adapter\"" w677 {
          tunnel: [_ "UpdateInterfaceMethods"] -> w676
          frame "Parent", Default {
          }
          frame "Adapter" {
          }
        }
      }
      frame "UpdateInterfaceMethods" {
        n269 = local read "MyClassMethods(Interface)"() -> (w735:i32[])
        n270 = property on="MyClassMethods(Interface)" class="LstBox (strict)" props=["Item Names", "Item Symbols"]() -> ("Item Names"=w739:string[])  [unwired: 2 in, 3 out]
        n271 = for {
          tunnel: w739 -> [_] mode=indexing
          tunnel: [w744] -> w738 mode=indexing if=w742
          tunnel: w735 -> [w745]
          i -> [w744]
          n272 = Search 1D Array(1D array=w745, element=w744) -> (index of element=w743:i32)  [unwired: 1 in]
          n273 = Less Than 0?(x=w743) -> (x < 0?=w742:bool)
        }
        n274 = Build Array(w739) -> (w741:string[][])
        n275 = Transpose 2D Array(2D array=w741) -> (transposed array=w740:string[][])
        n276 = property on="Parent Methods" class="MCListbox (strict)"("ItemNames"=w740, "DisabledItems"=w738) -> ()  [unwired: 2 in, 2 out]
      }
      frame "UpdateCP" {
        w762 = u32[] []
        # "444=4815\n565=4833\n686=4834"
        n277 = Unbundle By Name(w765) -> ("Classes"=w764:refnum<vi>[], "Selected"=w763:i32[])
        n278 = for {
          tunnel: w764 -> [w785]
          tunnel: w763 -> [w784] mode=indexing
          shift-right: [w778] -> w761
          shift-left: w762 -> [w779]
          shift-right: [w776] -> w755
          shift-left: w762 -> [w777]
          n279 = Index Array(array=w785, index=w784) -> (element=w783:refnum<vi>)
          n280 = property class="LVClassLibrary"(reference=w783) -> ("Dynamic Member VIs"=w782:refnum<vi>[], "Static Member VIs"=w781:refnum<vi>[])  [unwired: 1 in, 2 out]
          n281 = Build Array (concatenate)(w782, w781) -> (w780:refnum<vi>[])
          n282 = for {
            tunnel: w780 -> [w795] mode=indexing
            shift-right: [w788] -> w778
            shift-left: w779 -> [w790]
            shift-right: [w786] -> w776
            shift-left: w777 -> [w787]
            n283 = property class="VI"(reference=w795) -> (reference out=w792:refnum<vi>, "ConPane"=w794:refnum<vi>)  [unwired: 1 in, 1 out]
            n284 = property class="ConPane"(reference=w794) -> (error out=w793:errorcluster, "Pattern"=w789:u32)  [unwired: 1 in, 1 out]
            n285 = Search 1D Array(1D array=w790, element=w789) -> (index of element=w791:i32)  [unwired: 1 in]
            n286 = case shown="-1" w791 {
              selector: w791 -> [w796 _]
              tunnel: w790 -> [w799 w806]
              tunnel: w789 -> [_ w807]
              tunnel: [w799 w805] -> w788
              tunnel: w787 -> [w798 w803]
              tunnel: [w797 w802] -> w786
              frame 0, Default {
                n287 = in-place {
                  n288 = in-place-array #2(w798, w796) -> (w801:u32)
                  n289 = Increment(x=w801) -> (x+1=w800:u32)
                  n290 = in-place-array #2(w800) -> (w797:u32[])  [unwired: 1 out]
                }
              }
              frame -1 {
                n291 = Build Array (concatenate)(w806, w807) -> (w805:u32[])
                n292 = Build Array (concatenate)(w803, u32 1 ("Pattern")) -> (w802:u32[])
              }
            }
            n293 = Close Reference(reference=w792, error in (no error)=w793) -> ()  [unwired: 1 out]
          }
        }
        n294 = Array Size(array=w755) -> (size(s)=w754:i32)
        n295 = Array Max & Min(array=w755) -> (max index (indices)=w760:i32)  [unwired: 3 out]
        n296 = Index Array(array=w761, index=w760) -> (element=w759:u32)
        n297 = Greater?(x=w754, y=1) -> (0:w750:bool)
        n298 = case shown="4815, Default" w759 {
          tunnel: [w769 w772 w775] -> w756
          tunnel: [0 1 2] -> w752
          tunnel: [w767 w771 w774] -> w751
          frame 4815, Default {
            w767 = u16 2 items=["4x4x4", "5x6x5", "6x8x6"] ("CP2")
            w769 = T1 0 items=["4x4x4", "5x6x5", "6x8x6"] ("CP1")
          }
          frame 4833 {
            w771 = u16 2 items=["4x4x4", "5x6x5", "6x8x6"] ("CP2")
            w772 = T1 1 items=["4x4x4", "5x6x5", "6x8x6"] ("CP1")
          }
          frame 4834 {
            w774 = u16 0 items=["4x4x4", "5x6x5", "6x8x6"] ("CP2")
            w775 = T1 2 items=["4x4x4", "5x6x5", "6x8x6"] ("CP1")
          }
        }
        n299 = Select(t=T4."Disabled and Grayed Out", s=w750, f=T4."Enabled" ("Disabled")) -> (s? t:f=w746:T4)
        n300 = property on="CP1" class="Ring (strict)"("Value"=w756, "DisabledEnum"=w746) -> ()  [unwired: 2 in, 2 out]
        n301 = Build Array(w752) -> (w749:i32[])
        n302 = Select(t=i32[] [], s=w750, f=w749) -> (s? t:f=w748:i32[])
        n303 = property on="CP2" class="Ring (strict)"("Disabled Items []"=w748, "Value"=w751) -> ()  [unwired: 2 in, 2 out]
      }
      frame "", "Idle" {
        n304 = event shown="[6] \"Class(es)\": Value Change" {
          selector: _ -> [_ _ _ _ _ _ _ _ _ _ _ _ _ _ _ _]
          dyn-events: _ -> [_ _ _ _ _ _ _ _ _ _ _ _ _ _ _ _]
          timeout: 100 -> [_ _ _ _ _ _ _ _ _ _ _ _ _ _ _ _]
          tunnel: w811 -> [w823 w833 w834 w838 w842 w854 w876 w899 w906 w921 w940 w945 w947 w948 w954 w971]
          tunnel: [w821 w833 w834 w838 w842 w854 w874 w899 w906 w921 w940 w945 w947 w948 w953 w971] -> w816
          tunnel: ["Update" "ApplyCp" "Exit" "UpdateClassControl" w840 "Idle" "Update" _ "UpdateInterfaceTab" "UpdateInterfaceTab" w931 "UpdateInterfaceTab" "UpdateInterfaceMethods" _ _ "UpdateClassControlNames"] -> w815
          tunnel: w813 -> [w825 _ _ _ _ w857 _ _ _ _ _ _ _ _ _ _]
          tunnel: w812 -> [w824 _ _ _ _ w856 _ _ _ _ _ _ _ _ _ _]
          tunnel: w811 -> [w820 _ _ _ _ _ _ w898 _ _ _ _ _ _ _ _]
          tunnel: w810 -> [_ _ _ _ _ _ _ _ w904 w919 _ _ _ _ _ _]
          tunnel: w808 -> [_ _ _ _ _ _ _ _ w901 w917 _ _ _ _ _ _]
          event "ClassesOK", "ClassesCancel": Value Change {
            n305 = event-data() -> ()  [unwired: 1 in, 1 out]
            n306 = Unbundle By Name(w820) -> ("Selected"=w818:i32[])
            n307 = case shown="True" "ClassesOK" {
              tunnel: w818 -> [w826 _]
              tunnel: [w826 w827] -> w817
              frame False {
                n308 = local write "Classes"(w826) -> ()
              }
              frame True {
                n309 = local read "Classes"() -> (w827:i32[])
              }
            }
            n310 = for {
              tunnel: w825 -> [w831] mode=indexing
              n311 = property on="Property Node" class="Ctl"(reference=w831, "Visible"=FALSE) -> ()  [unwired: 1 in, 2 out]
            }
            n312 = for {
              tunnel: w824 -> [w829] mode=indexing
              n313 = property on="Property Node" class="Ctl"(reference=w829, "Visible"=TRUE) -> ()  [unwired: 1 in, 2 out]
            }
            n314 = Bundle By Name(cluster=w823, "Selected"=w817) -> (w821:T2)
          }
          event "ApplyCP": Value Change {
            n315 = event-data() -> ()  [unwired: 1 in, 6 out]
          }
          event Panel Close? {
            n316 = event-data() -> ()  [unwired: 1 in, 1 out]
            n317 = event-data("Discard?"=TRUE) -> ()  [unwired: 1 in, 1 out]
          }
          event "ClassControlName": Value Change {
            n318 = event-data() -> ()  [unwired: 1 in, 2 out]
          }
          event "Tab": Value Change {
            n319 = event-data() -> ()  [unwired: 1 in, 2 out]
            n320 = case shown="\"Interface\"" "Tab" {
              tunnel: ["UpdateCP" "UpdateClassControl" "CheckClassSelection"] -> w840
              tunnel: [TRUE TRUE _] -> w839
              frame "CP", Default {
              }
              frame "ClassControlName" {
              }
              frame "Interface" {
              }
            }
            n321 = property on="MoreClasses" class="Bool"("Visible"=w839) -> ()  [unwired: 2 in, 2 out]
          }
          event "MoreClasses": Value Change {
            n322 = event-data() -> ()  [unwired: 1 in, 2 out]
            n323 = local read "Classes"() -> (w853:i32[])
            n324 = property on="Classes" class="LstBox (strict)"() -> ("Top Row"=w850:i32)  [unwired: 2 in, 2 out]
            n325 = Index Array(array=w853) -> (element=w848:i32)  [unwired: 1 in]
            n326 = for {
              tunnel: w857 -> [w862] mode=indexing
              n327 = property on="Property Node" class="Ctl"(reference=w862, "Visible"=TRUE) -> ()  [unwired: 1 in, 2 out]
            }
            n328 = for {
              tunnel: w856 -> [w860] mode=indexing
              n329 = property on="Property Node" class="Ctl"(reference=w860, "Visible"=FALSE) -> ()  [unwired: 1 in, 2 out]
            }
            n330 = Add(x=w850, y=32) -> (x+y=w851:i32)
            n331 = In Range and Coerce(upper limit=w851, x=w848, lower limit=w850) -> (In Range?=w849:bool)  [unwired: 1 out]
            n332 = case shown="False" w849 {
              tunnel: w848 -> [w858 _]
              frame False {
                n333 = property on="Classes" class="LstBox (strict)"("Top Row"=w858) -> ()  [unwired: 2 in, 2 out]
              }
              frame True {
              }
            }
          }
          event "Class(es)": Value Change {
            n334 = event-data() -> ()  [unwired: 1 in, 2 out]
            n335 = Subtract(x="Class(es)", y=u16 2) -> (x-y=w873:u16)
            n336 = case shown="0.." w873 {
              selector: w873 -> [_ w879]
              frame Default {
              }
              frame 0.. {
                n337 = property on="Classes" class="LstBox (strict)"() -> ("Item Names"=w882:string[])  [unwired: 2 in, 2 out]
                n338 = Index Array(array=w882, index=w879) -> (element=w883:string)
                n339 = Build Array (concatenate)(w883, "-" ("element"), w882) -> (w881:string[])
                n340 = property on="Class(es)" class="Ring (strict)"("Strings []"=w881, "Value"=0 ("Classes")) -> ()  [unwired: 2 in, 2 out]
              }
            }
            n341 = Build Array(w873) -> (w872:u16[])
            n342 = property on="Classes" class="LstBox (strict)"("Value"=w872) -> ()  [unwired: 2 in, 2 out]
            n343 = property on="ParentFolder" class="Path"("DisabledEnum"=T4."Enabled" ("Disabled")) -> ()  [unwired: 2 in, 2 out]
            n344 = local write "ParentClass"(0 ("Classes")) -> ()
            n345 = local write "ParentFolder"(path "" ("ParentFolder")) -> ()
            n346 = Bundle By Name(cluster=w876, "Selected"=w872) -> (w874:T2)
            n347 = property on="MyClassMethods(Interface)" class="LstBox (strict)"("Item Names"=string[] [], "Value"=i32[] [] ("MyClassMethods")) -> ()  [unwired: 2 in, 2 out]
            n348 = local write "ParentClassName"("" ("Caption.Text")) -> ()
            n349 = property on="MyClassMethods" class="LstBox (strict)"("Item Names"=string[] [], "Value"=i32[] [] ("MyClassMethods")) -> ()  [unwired: 2 in, 2 out]
            n350 = property on="Class(es)" class="Ring (strict)"("Caption.Text"="") -> ()  [unwired: 2 in, 2 out]
          }
          event "ParentClass": Value Change {
            n351 = event-data() -> ()  [unwired: 1 in, 2 out]
            n352 = property on="ParentClass" class="Ring (strict)"() -> ("Strings []"=w896:string[])  [unwired: 2 in, 2 out]
            n353 = Unbundle By Name(w898) -> ("DropDownClasses"=w897:refnum<vi>[])
            n354 = Index Array(array=w896, index="ParentClass") -> (element=w893:string)
            n355 = Decrement(x="ParentClass") -> (x-1=w886:u16)
            n356 = Index Array(array=w897, index=w886) -> (element=w892:refnum<vi>)
            n357 = property class="LVClassLibrary"(reference=w892) -> ("Path"=w885:path)  [unwired: 1 in, 2 out]
            n358 = Strip Path(path=w885) -> (stripped path=w891:path)  [unwired: 1 out]
            n359 = Empty String/Path?(string/path=w885) -> (empty?=w890:bool)
            n360 = Select(t=T4."Enabled" ("Disabled"), s=w890, f=T4."Disabled and Grayed Out" ("Disabled")) -> (s? t:f=w887:T4)
            n361 = property on="ParentFolder" class="Path"("Value"=w891, "DisabledEnum"=w887) -> ()  [unwired: 2 in, 2 out]
            n362 = property on="ParentClassName" class="Str"("Text.TextColor"=u32 0, "Value"=w893, "DisabledEnum"=w887) -> ()  [unwired: 2 in, 2 out]
          }
          event "ParentClassName": Value Change; "ParentClassName": Mouse Down {
            n363 = event-data() -> ("Type"=w905:T11)  [unwired: 1 in, 1 out]
            n364 = case shown="\"Mouse Down\"" w905 {
              tunnel: w904 -> [_ w913]
              tunnel: "ParentClassName" -> [_ w910]
              tunnel: w901 -> [_ w911]
              frame "Null", Default {
              }
              frame "Mouse Down" {
                n365 = Equal?(x=w913, y=w910) -> (x = y?=w907:bool)
                n366 = Equal?(x=w911, y=w910) -> (x = y?=w908:bool)
                n367 = Or(x=w907, y=w908) -> (x .or. y?=w909:bool)
                n368 = property on="ParentClassName" class="Str"("Key Focus"=TRUE) -> ()  [unwired: 2 in, 2 out]
                n369 = case shown="True" w909 {
                  frame False {
                  }
                  frame True {
                    n370 = local write "ParentClassName"("" ("ParentClassName")) -> ()
                  }
                }
              }
            }
            n371 = property on="ParentClassName" class="Str"("Text.TextColor"=u32 0) -> ()  [unwired: 2 in, 2 out]
          }
          event "InterfaceClassName": Mouse Down; "InterfaceClassName": Value Change {
            n372 = event-data() -> ("Type"=w920:T11)  [unwired: 1 in, 1 out]
            n373 = case shown="\"Null\", Default" w920 {
              tunnel: w919 -> [_ w928]
              tunnel: "InterfaceClassName" -> [_ w925]
              tunnel: w917 -> [_ w926]
              frame "Null", Default {
              }
              frame "Mouse Down" {
                n374 = Equal?(x=w928, y=w925) -> (x = y?=w922:bool)
                n375 = Equal?(x=w926, y=w925) -> (x = y?=w923:bool)
                n376 = Or(x=w922, y=w923) -> (x .or. y?=w924:bool)
                n377 = property on="InterfaceClassName" class="Str"("Key Focus"=TRUE) -> ()  [unwired: 2 in, 2 out]
                n378 = case shown="True" w924 {
                  frame False {
                  }
                  frame True {
                    n379 = local write "InterfaceClassName"("" ("ParentClassName")) -> ()
                  }
                }
              }
            }
            n380 = property on="InterfaceClassName" class="Str"("Text.TextColor"=u32 0) -> ()  [unwired: 2 in, 2 out]
          }
          event Timeout {
            n381 = event-data() -> ()  [unwired: 1 in, 3 out]
            n382 = local read "InterfaceOptionTab"() -> (w939:enum32{"Parent", "Adapter"})
            n383 = local read "ParentClassName"() -> (w937:string)
            n384 = local read "InterfaceToCreate"() -> (w936:u16)
            n385 = Less Or Equal?(x=w936, y=u16 1 ("Classes")) -> (x <= y?=w932:bool)
            n386 = Empty String/Path?(string/path=w937) -> (empty?=w934:bool)
            n387 = Equal?(x=w939, y=enum32{"Parent", "Adapter"}."Parent" ("InterfaceOptionTab")) -> (x = y?=w933:bool)
            n388 = Compound Arithmetic op=AND(w934, w933, w932) -> (w930:bool)
            n389 = case shown="True" w930 {
              tunnel: [_ "UpdateInterfaceTab"] -> w931
              frame False {
              }
              frame True {
              }
            }
          }
          event "InterfaceToCreate": Value Change {
            n390 = event-data() -> ()  [unwired: 1 in, 6 out]
            n391 = local write "ParentClassName"("" ("ParentClassName")) -> ()
            n392 = local write "ParentFolder"(path "" ("ParentFolder")) -> ()
          }
          event "MyClassMethods(Interface)": Value Change {
            n393 = event-data() -> ()  [unwired: 1 in, 6 out]
          }
          event "SelectAll": Value Change {
            n394 = event-data() -> ()  [unwired: 1 in, 2 out]
            n395 = property on="Classes" class="LstBox (strict)"() -> ("Item Names"=w951:string[])  [unwired: 2 in, 2 out]
            n396 = Array Size(array=w951) -> (size(s)=w950:i32)
            n397 = for {
              N: w950 -> [_]
              tunnel: [w952] -> w949 mode=indexing
              i -> [w952]
            }
            n398 = property on="Classes" class="LstBox (strict)"("Value"=w949) -> ()  [unwired: 2 in, 2 out]
          }
          event Key Down {
            n399 = event-data() -> ("Char"=w957:i16, "PlatMods.Ctrl"=w958:bool)  [unwired: 1 in]
            n400 = property on="Classes" class="LstBox (strict)"() -> ("Visible"=w955:bool)  [unwired: 2 in, 2 out]
            n401 = And(x=w958, y=w955) -> (x .and. y?=w956:bool)
            n402 = case shown="True" w956 {
              tunnel: w957 -> [_ w962]
              tunnel: w954 -> [w959 w961]
              tunnel: [w959 w960] -> w953
              frame False {
              }
              frame True {
                n403 = case shown="65, 97" w962 {
                  tunnel: w961 -> [w963 w966]
                  tunnel: [w963 w965] -> w960
                  frame 0, Default {
                  }
                  frame 65, 97 {
                    n404 = property on="Classes" class="LstBox (strict)"() -> ("Item Names"=w968:string[])  [unwired: 2 in, 2 out]
                    n405 = Array Size(array=w968) -> (size(s)=w967:i32)
                    n406 = for {
                      N: w967 -> [_]
                      tunnel: [w969] -> w964 mode=indexing
                      i -> [w969]
                    }
                    n407 = property on="Classes" class="LstBox (strict)"("Value"=w964) -> ()  [unwired: 2 in, 2 out]
                    n408 = Bundle By Name(cluster=w966, "Selected"=w964) -> (w965:T2)
                  }
                }
              }
            }
          }
          event "UpdateClassControlNames": Value Change {
            n409 = event-data() -> ()  [unwired: 1 in, 6 out]
          }
        }
      }
      frame "CheckClassSelection" {
        n410 = Unbundle By Name(w976) -> ("Selected"=w978:i32[])
        n411 = Index Array(array=w978) -> (element=w977:i32)  [unwired: 1 in]
        n412 = Build Array(w977) -> (w975:i32[])
        n413 = Bundle By Name(cluster=w976, "Selected"=w975) -> (w974:T2)
      }
      frame "UpdateClassControlNames" {
        n414 = Unbundle By Name(w983) -> ("Classes"=w985:refnum<vi>[], "Selected"=w984:i32[])
        n415 = local read "ClassControlName"() -> (w979:string)
        n416 = for {
          tunnel: w985 -> [w991]
          tunnel: w984 -> [w987] mode=indexing
          shift-right: [w989] -> w981
          shift-left: w982 -> [w988]
          tunnel: w979 -> [w986]
          n417 = Index Array(array=w991, index=w987) -> (element=w990:refnum<vi>)
          n418 = disable-structure shown="Disabled" {
            disable-tunnel: w990 -> [w995 _]
            disable-tunnel: [w994 _] -> w989
            disable-tunnel: w988 -> [w993 _]
            disable-tunnel: w986 -> [w992 _]
            frame Disabled {
              n419 = call <resource>:"Scripting_RenameClassControlsOfClass.vi"("error in (no error)"=w993, "ClassControlName"=w992, "LVClassLibrary in"=w995) -> ("error out"=w994:errorcluster)  [unwired: 8 in]
            }
            frame Enabled {
            }
          }
        }
      }
      frame "ApplyCp" {
        n420 = call <vilib>:"Set Busy.vi"("error in (no error)"=w1000) -> ("error out"=w998:errorcluster)  [unwired: 9 in, 1 out]
        n421 = case shown="2, Default" "CP2" {
          tunnel: [w1022 w1023 w1024] -> w996
          frame 0 {
            w1022 = T1 0 items=["4x4x4", "5x6x5", "6x8x6"] ("Pattern")
          }
          frame 1 {
            w1023 = T1 1 items=["4x4x4", "5x6x5", "6x8x6"] ("Pattern")
          }
          frame 2, Default {
            w1024 = T1 2 items=["4x4x4", "5x6x5", "6x8x6"] ("Pattern")
          }
        }
        n422 = Unbundle By Name(w1003) -> ("Classes"=w1002:refnum<vi>[], "Selected"=w1001:i32[])
        n423 = for {
          shift-right: [w1011] -> w999
          shift-left: w998 -> [w1021]
          tunnel: w1002 -> [w1020]
          tunnel: w1001 -> [w1019] mode=indexing
          tunnel: w996 -> [w1007]
          n424 = Index Array(array=w1020, index=w1019) -> (element=w1018:refnum<vi>)
          n425 = call <resource>:"GDSLvClass_ReadClassType.vi"("Class Refnum In"=w1018, "error in (no error)"=w1021) -> ("Class Refnum Out"=w1014:refnum<vi>, "ClassSettings"=w1009:T6, "error out"=w1015:errorcluster)  [unwired: 15 in]
          n426 = Unbundle By Name(w1009) -> ("ClassTemplateUsed"=w1008:string)
          n427 = call "GOOP_TemplateRename.vi"("Ring"=w1007, "TemplateIn"=w1008) -> ("TemplateOut"=w1006:string)  [unwired: 9 in]
          n428 = Format Into String(w1007) -> (resulting string=w1010:string)  [unwired: 3 in, 1 out]
          n429 = Bundle By Name(cluster=w1009, "ConnectorPanePattern"=w1010, "ClassTemplateUsed"=w1006) -> (w1017:T6)
          n430 = call <resource>:"GDSLvClass_StoreClassType.vi"("Class Refnum In"=w1014, "ClassSettings"=w1017, "CheckAndFixConnectorPaneType(False)"=TRUE, "error in (no error)"=w1015) -> ("Class Refnum Out"=w1013:refnum<vi>, "error out"=w1012:errorcluster)  [unwired: 14 in]
          n431 = invoke class="LVClassLibrary" method="Save"(reference=w1013, error in=w1012) -> (error out=w1011:errorcluster)  [unwired: 2 in, 3 out]
        }
        n432 = call <vilib>:"Unset Busy.vi"("error in (no error)"=w999) -> ("error out"=w997:errorcluster)  [unwired: 10 in]
      }
      frame "UpdateClassControl" {
        n433 = local read "ClassControlName"() -> (w1037:string)
        n434 = Unbundle By Name(w1041) -> ("Selected"=w1039:i32[])
        n435 = Index Array(array=w1039) -> (element=w1038:i32)  [unwired: 1 in]
        n436 = property on="Classes" class="LstBox (strict)"() -> ("Item Names"=w1040:string[])  [unwired: 2 in, 2 out]
        n437 = Index Array(array=w1040, index=w1038) -> (element=w1035:string)
        n438 = Search and Replace String(case sensitive?=TRUE ("ignore case? (F)"), input string=w1037, search string="<ClassName>" ("substring (\"\")"), replace string=w1035) -> (result string=w1033:string)  [unwired: 4 in, 3 out]
        n439 = xnode "Match Regular Expression"("input string"=w1033, "regular expression"="(\\w+)/(\\w+)") -> ("before match"=w1030:string, "after match"=w1028:string, "offset past match"=w1031:i32, "submatch 1"=w1029:string, "submatch 2"=w1027:string)  [unwired: 4 in, 2 out]
        n440 = case shown="0, Default" w1031 {
          tunnel: w1030 -> [w1047 w1049]
          tunnel: w1029 -> [w1048 _]
          tunnel: w1028 -> [w1045 _]
          tunnel: w1027 -> [w1046 _]
          tunnel: [w1044 w1049] -> w1026
          tunnel: [w1043 w1049] -> w1025
          frame 0, Default {
            n441 = Concatenate Strings(w1047, w1048, w1045) -> (w1044:string)
            n442 = Concatenate Strings(w1047, w1046, w1045) -> (w1043:string)
          }
          frame -1 {
          }
        }
        "ClassNameIn" <- w1026
        "ClassNameOut" <- w1025
      }
    }
    n443 = Select(t="Error", s=w41, f=w42) -> (s? t:f=w44:string)
  }
  "Error Out" <- w24
  n444 = Unbundle By Name(w12) -> ("Classes"=w11:refnum<vi>[])
  n445 = Close Reference(reference=w11) -> ()  [unwired: 1 in, 1 out]
